vi "MotorVelocity_To_SteeringFrameVelocity(SubVI).vi"(11 "ccw motor velocity states":dbl[](array[numeric])) -> (2 "rotation_velocity":dbl, 3 "forward_velocity":dbl)   [LabVIEW 2017]
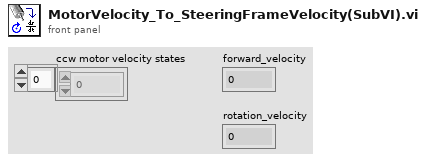
[diagram p1: front panel]
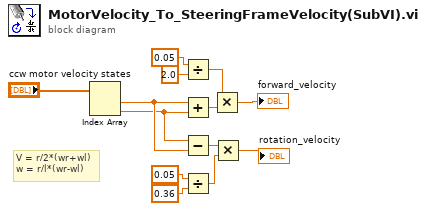
[diagram p0: block diagram]
diagram:
  # "V = r/2*(wr+wl)\nw = r/l*(wr-wl)"
  n1 = Index Array(array="ccw motor velocity states") -> (element #1=w8:dbl, element #2=w7:dbl)  [unwired: 2 in]
  n2 = Divide(x=0.05, y=2.0) -> (x/y=w5:dbl)
  n3 = Add(x=w8, y=w7) -> (x+y=w2:dbl)
  n4 = Subtract(x=w7, y=w8) -> (x-y=w9:dbl)
  n5 = Divide(x=0.05, y=0.36) -> (x/y=w10:dbl)
  n6 = Multiply(x=w5, y=w2) -> (x*y=→"forward_velocity":dbl)
  n7 = Multiply(x=w9, y=w10) -> (x*y=→"rotation_velocity":dbl)
